vi "Measure vs B2Dv3.vi"() -> ()   [LabVIEW 2009]
doc: "This VI is an example operator panel.\n\nThe VI contains a table for the field values that may be configured manually, or loaded by checking the \"Prompt for File\" box. The data file should contain 3 columns of data, with each column delimited by a tab character.\n\nBefore the VI is executed, set the desired field units and coordinate system. Once the VI is started, follow the directions in the STATUS indicator to operate. Once a field value is achieved, it will be held indefinitely with no user intervention.\n\nThe present field is displayed in the selected units and coordinate system. The present field is queried once per second.\n\nIf a field point is specified that is outside the limits for the magnet, the VI will abort execution."
uses:
  <vilib>/Utility/file.llb/Read From Spreadsheet File (DBL).vi
panel:
  in  "FieldRange":dbl=1.0
  in  "Change\nPID\n(DetermineSIMPID.vi)":bool
  in  "Wait between \nVectors (ms)":u32=4000
  in  "X Axis":enum16{"B", "phi"}(ring)
  in  "Y Axis":T1(ring)=enum."HP (V)"
  out "measured data":dbl[][](array[numeric])
  out "XY Graph":T2(graph)
  in  "Notes:":string="Datum: 22.08.11, Uhrzeit: 18:21, T`0.3K, PID LOOP: P -0.2 I 200 D off, PID Dämpfung: P0,4 D2.2E-5, Laser 25°, 20mA, AOM 10mA, Sweep 0.15T/min " caption="Notizen:"
  out "Messfile Refnum":refnum<file>
  in  "Measurement File":path=path "D:/UserData/Matthias/Messungen/STO_LAOR103/110822/110822_R103_0deg_-0.4--9T_2.txt"
  in  "Sample name:":string="R103"
  in  "HP 1":bool=TRUE
  in  "GPIB HP":string="14"
  in  "LI 4":bool
  in  "GPIB L 4":string="8"
  in  "LI 3":bool
  in  "GPIB L 3":string="8"
  in  "LI 2":bool
  in  "GPIB L 2":string="8"
  in  "LI 1":bool
  in  "GPIB L 1":string="8"
  out "Number of lines":i32=1
  in  "Operation":u16(ring)=1 items=["Stepwise", "Continous"]
  out "Ramp Rate along Vector (T/min)":dbl=0.15000000000000002 format="%.3f"
  out "Current Ramp Rate Z (T/min)":dbl=0.15000000000000002 format="%.3f"
  out "Current Ramp Rate Y (T/min)":dbl format="%.3f"
  in  "User defined Ramp Rate (T/min)":bool=TRUE
  in  "User defined Ramp Rate (T/min)":dbl=0.15 format="%.3f"
  in  "Z-Axis Communications Config":T3={"GPIB address"=22, "GPIB bus"=1, "connection ID"=refnum, "IP"="111.111.111.1", "Active Comm Interface"=0, "Serial Port"="", "Programmer Type"=0} {"Programmer Type" items=["Model 430", "Model 420"]; "Active Comm Interface" items=["TCP/IP (Model 430 Only)", "RS232", "IEEE488"]}
  in  "Max Ramp Rate - Y Axis (A/s)":dbl=0.065 format="%.3f"
  in  "Max Ramp Rate - Z Axis (A/s)":dbl=0.203 format="%.3f"
  in  "Magnitude Limit (kG)":dbl=45.1 format="%.3f"
  in  "Y-Axis Communications Config":T3={"GPIB address"=22, "GPIB bus"=1, "connection ID"=refnum, "IP"="111.111.111.2", "Active Comm Interface"=0, "Serial Port"="", "Programmer Type"=0} {"Programmer Type" items=["Model 430", "Model 420"]; "Active Comm Interface" items=["TCP/IP (Model 430 Only)", "RS232", "IEEE488"]}
  out "Cartesian Display (T)":T4={"Y-Axis Field (T)"=-1e-05, "Z-Axis Field (T)"=-0.15342} {"Z-Axis Field (T)" format="%.3f"; "Y-Axis Field (T)" format="%.3f"}
  in  "Starting index":i32=1
  in  "Normal color":u32(colorbox)=11711154
  in  "Highlight color":u32(colorbox)=16711680
  in  "Prompt for File?":bool
  out "Continue Execution?":bool=TRUE
  out "error out":T5
  in  "error in":T5
  out "STATUS":string="Holding at current vector. Set Ramping Mode to NEXT VECTOR to continue."
  in  "Ramping Control":u16(ring)=2 items=["NEXT VECTOR", "RAMPING", "HOLDING", "PAUSE", "ZERO"]
  out "Cartesian Display (kG)":T6 {"Z-Axis Field (kG)" format="%.3f"; "Y-Axis Field (kG)" format="%.3f"}
  in  "Field Values":string[][](table)=[["0", "-0.4"]]
  out "Switch Heaters":bool=TRUE
  out "Polar Display (T)":T7={"q (degrees)"=90.0, "Field Magnitude (T)"=2e-05} {"Field Magnitude (T)" format="%.3f"; "q (degrees)" format="%.3f"}
  out "Polar Display (kG)":T8 {"Field Magnitude (kG)" format="%.3f"; "q (degrees)" format="%.3f"}
  in  "Coordinate System":u16(ring) items=["Cartesian", "Polar"]
  in  "Magnetic Field Units":u16(ring)=1 items=["kG", "Tesla"]
  # "Measurement Display"
  # "Measurement Settings"
  # "Magnet Settings"
  # "Max Ramp Rate z: 1.27 T/min\nMax Ramp Rate y: 0.17 T/min"
  # "Devices"
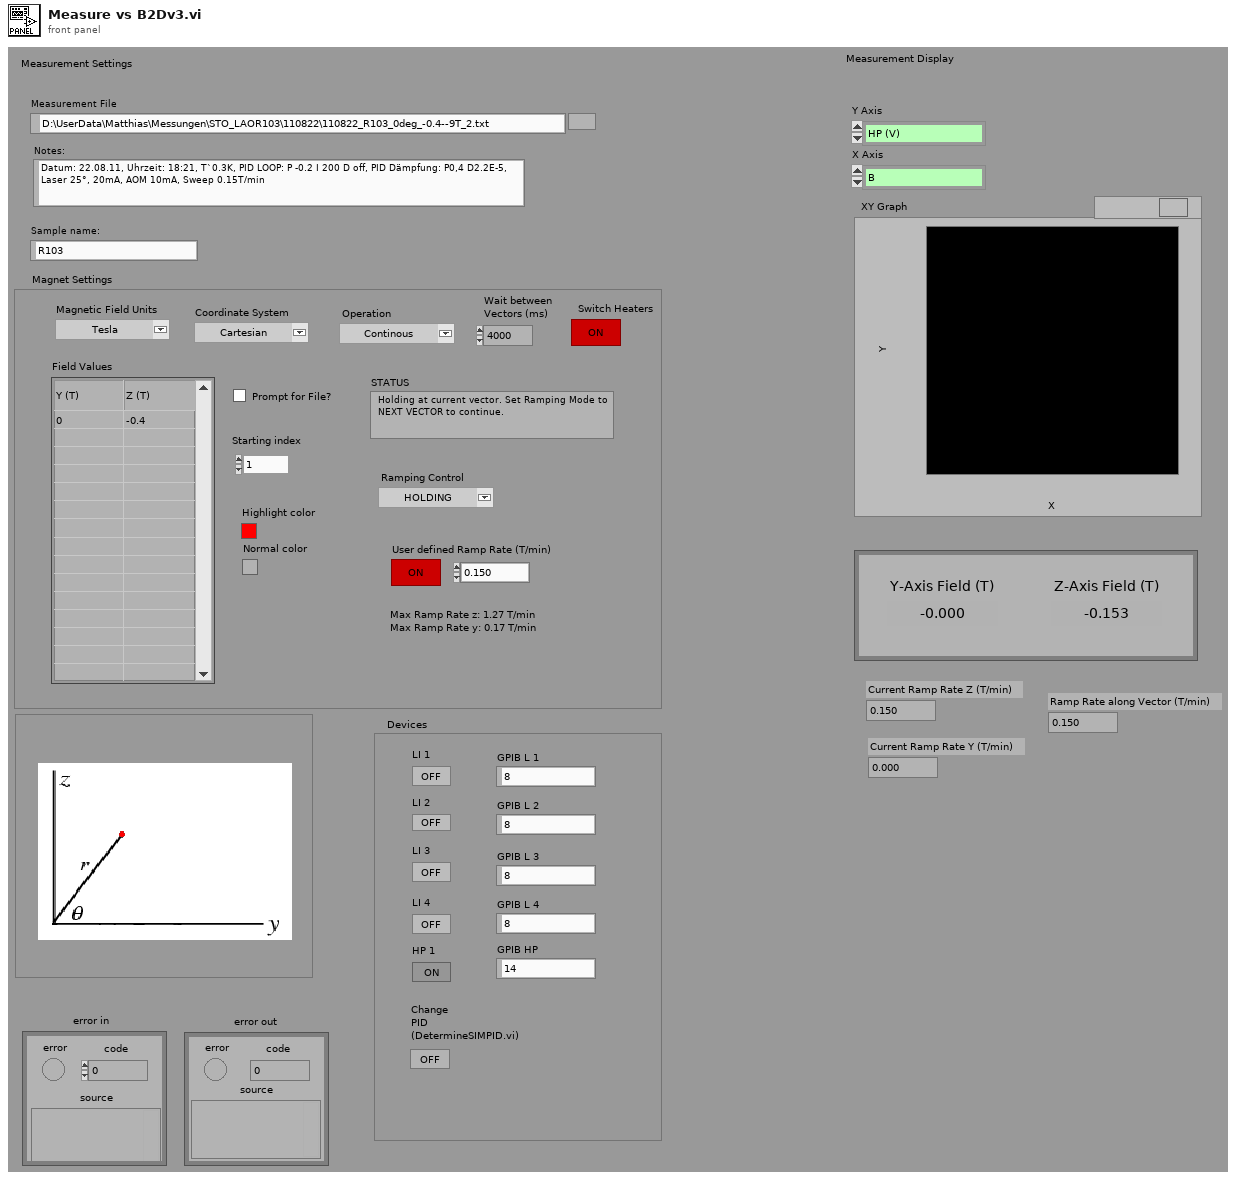
[diagram p1: front panel]
types:
  T1 = enum16{"B", "phi", "LI 1 Vx", "LI 1 phase", "LI 2 Vx", "LI 2 phase", "LI 3 Vx", "LI 3 phase", "LI 4 Vx", "LI 4 phase", "HP (V)"}
  T2 = cluster{"measured data":dbl[], "measured data":dbl[]}
  T3 = cluster{"GPIB address":i16, "GPIB bus":i16, "connection ID":refnum<k5>, "IP":string, "Active Comm Interface":u16, "Serial Port":refnum<visa-resource-name>, "Programmer Type":u16}
  T4 = cluster{"Y-Axis Field (T)":dbl, "Z-Axis Field (T)":dbl}
  T5 = cluster{"error":bool, "code":i32, "source":string}
  T6 = cluster{"Y-Axis Field (kG)":dbl, "Z-Axis Field (kG)":dbl}
  T7 = cluster{"q (degrees)":dbl, "Field Magnitude (T)":dbl}
  T8 = cluster{"q (degrees)":dbl, "Field Magnitude (kG)":dbl}
  T9 = enum16{"", "RAMPING", "HOLDING", "PAUSED", "MANUAL UP", "MANUAL DOWN", "ZEROING CURRENT", "QUENCH DETECTED", "HEATING SWITCH"}
  T10 = enum16{"", "RAMPING", "HOLDING", "PAUSED", "MANUAL UP", "MANUAL DOWN", "ZEROING CURRENT", "QUENCH DETECTED", "HEATING SWITCH", "AT ZER0", "COOLING SWITCH"}
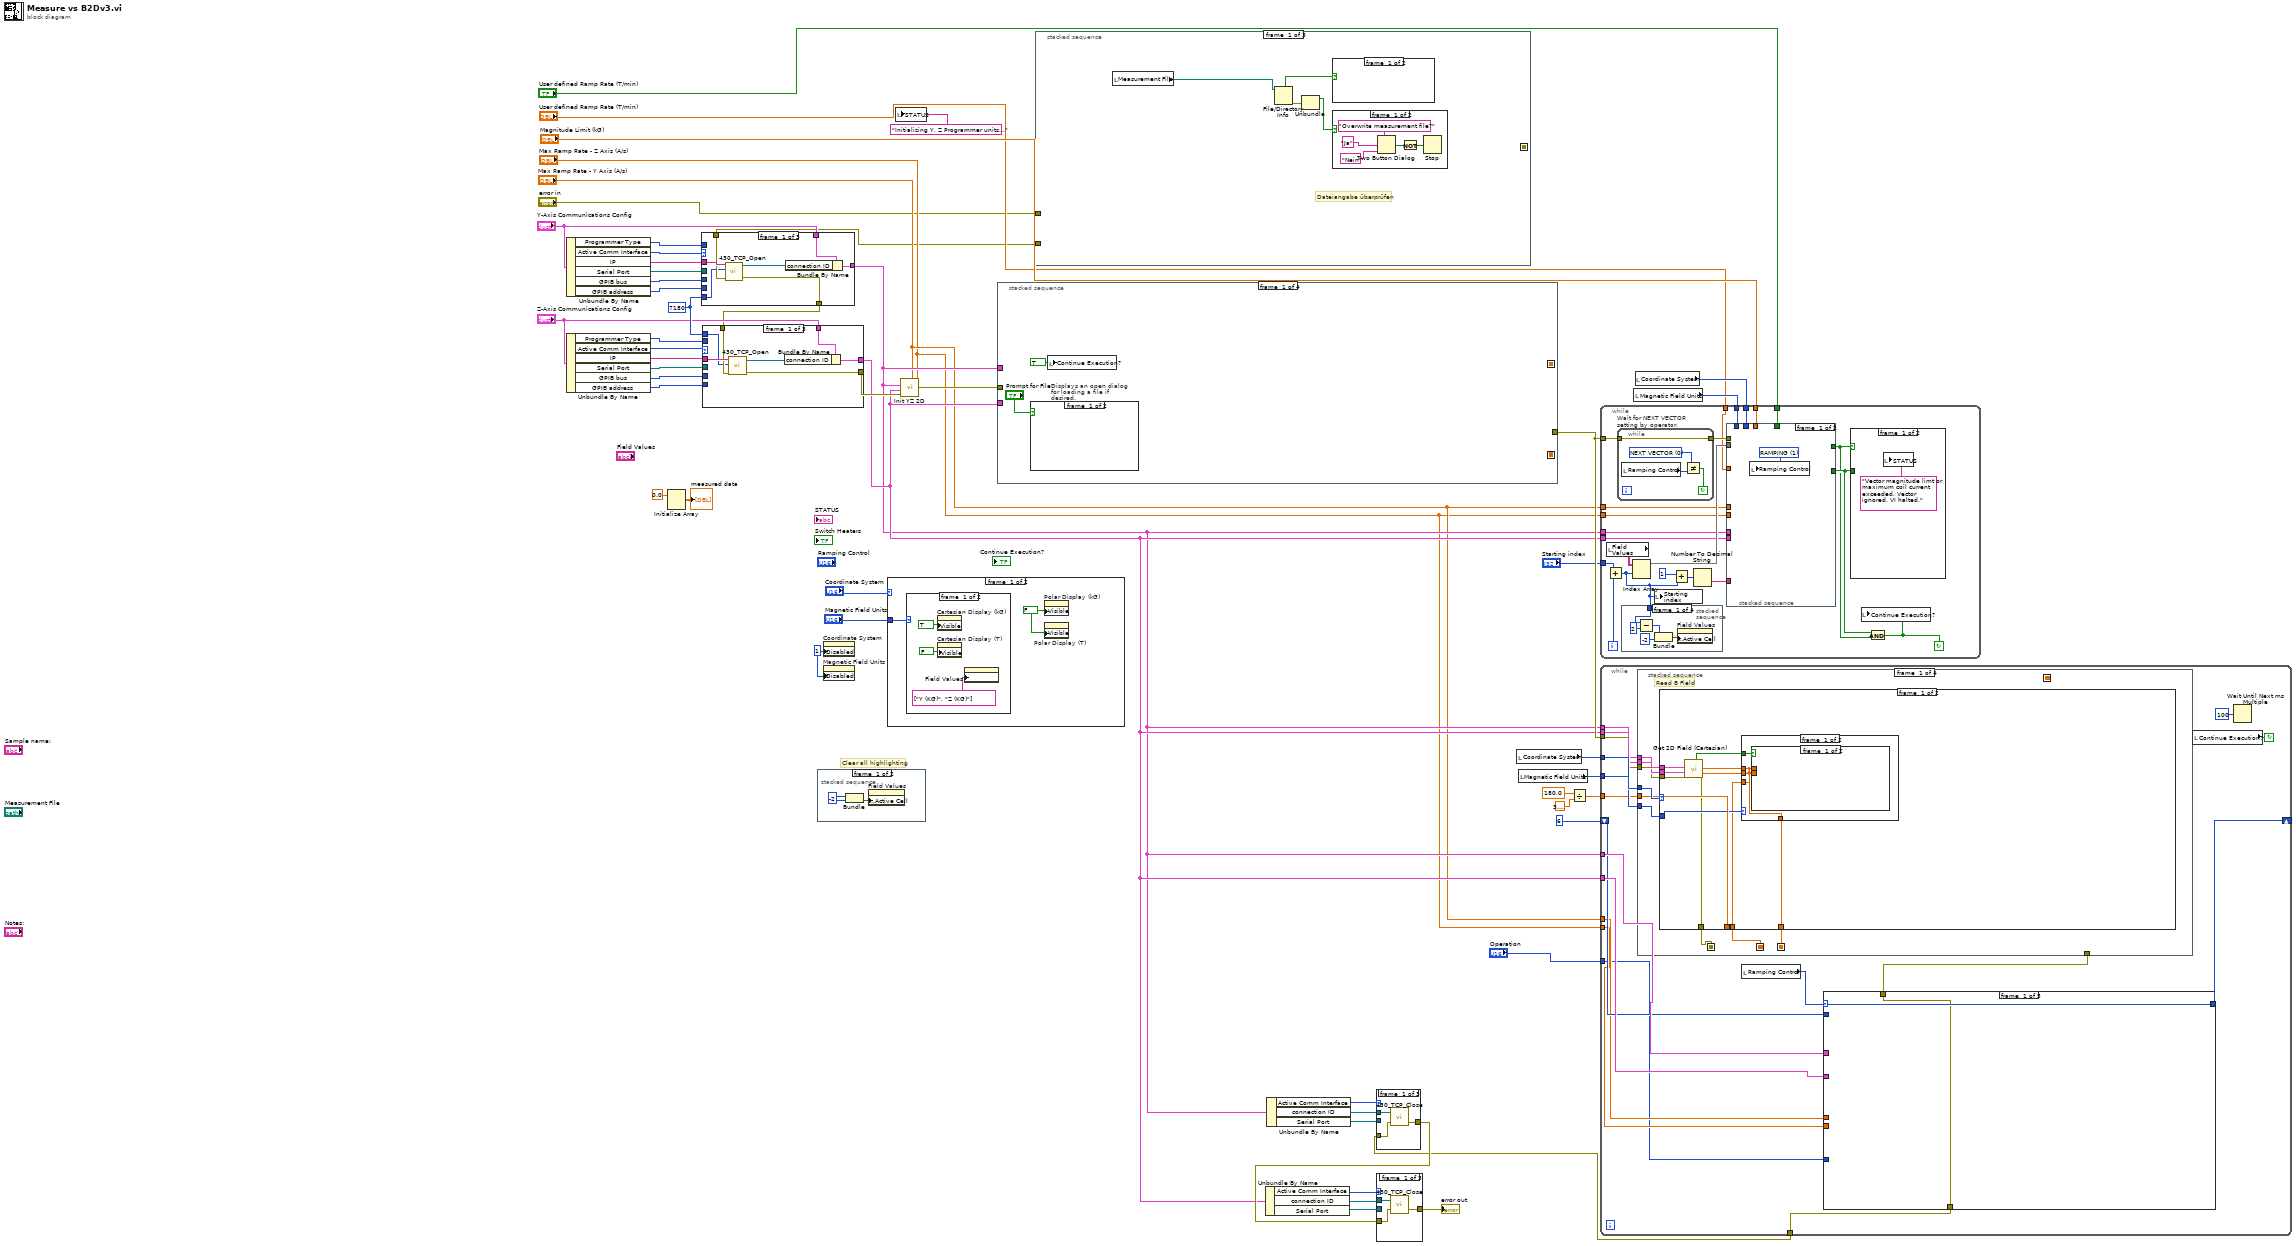
[diagram p0: block diagram]
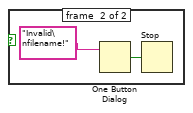
[diagram p3: hidden frame]
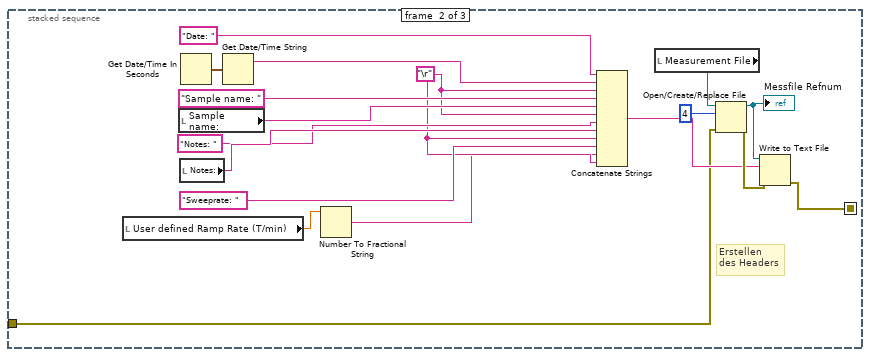
[diagram p4: hidden frame]
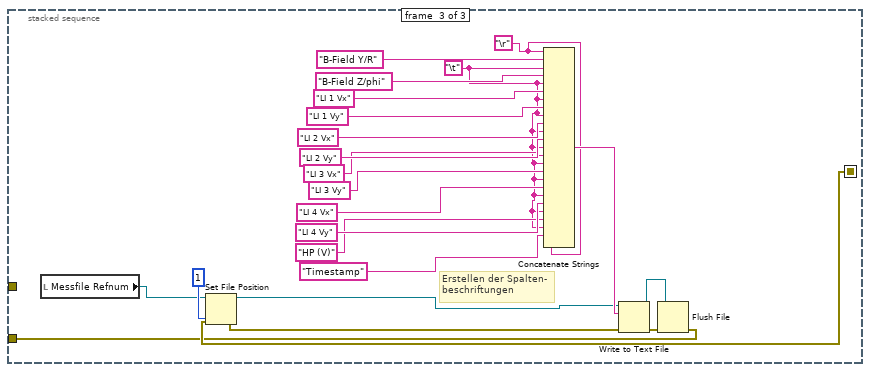
[diagram p5: hidden frame]
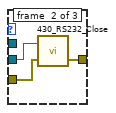
[diagram p6: hidden frame]
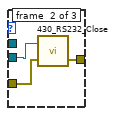
[diagram p8: hidden frame]
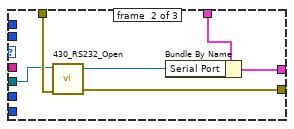
[diagram p10: hidden frame]
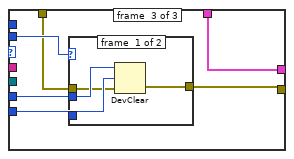
[diagram p11: hidden frame]
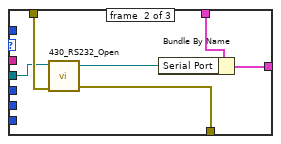
[diagram p13: hidden frame]
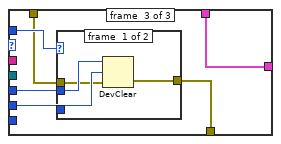
[diagram p14: hidden frame]
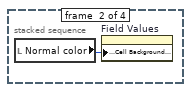
[diagram p16: hidden frame]
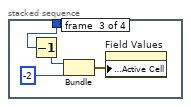
[diagram p17: hidden frame]
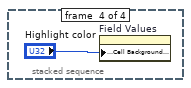
[diagram p18: hidden frame]
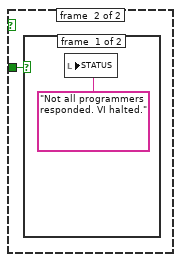
[diagram p19: hidden frame]
diagram:
  w38 = 7180 ("TCP Port")
  w51 = u8 1 ("Write Attribute")
  # "Clear all highlighting"
  n1 = Unbundle By Name("Z-Axis Communications Config") -> ("Programmer Type"=w14:u16, "Active Comm Interface"=w37:u16, "IP"=w34:string, "Serial Port"=w33:refnum<visa-resource-name>, "GPIB bus"=w13:i16, "GPIB address"=w12:i16)
  n2 = Unbundle By Name("Y-Axis Communications Config") -> ("Programmer Type"=w8:u16, "Active Comm Interface"=w36:u16, "IP"=w35:string, "Serial Port"=w32:refnum<visa-resource-name>, "GPIB bus"=w9:i16, "GPIB address"=w10:i16)
  n3 = Initialize Array(0.0 ("element")) -> (→"measured data":dbl[][])  [unwired: 2 in]
  n4 = stacked-sequence {
    frame #0 {
      w54 = -2
      n5 = Bundle(w54, w54) -> (w55:cluster{i32, i32})  [unwired: 1 in]
      n6 = property on="Field Values" class="Tbl (strict)"("Active Cell:Active Cell"=w55) -> ()  [unwired: 2 in, 2 out]
    }
    frame #1 {
      n7 = property on="Field Values" class="Tbl (strict)"("Active Cell:Cell Background Color"="Normal color") -> ()  [unwired: 2 in, 2 out]
    }
  }
  n8 = property on="Coordinate System" class="Ring (strict)"("Disabled"=w51) -> ()  [unwired: 2 in, 2 out]
  n9 = property on="Magnetic Field Units" class="Ring (strict)"("Disabled"=w51) -> ()  [unwired: 2 in, 2 out]
  n10 = case shown="0, Default" "Coordinate System" {
    tunnel: "Magnetic Field Units" -> [w58 w66]
    frame #0 {
      w57 = FALSE ("Write Attribute")
      (unwired) FALSE ("Write Attribute")
      (unwired) TRUE ("Write Attribute")
      n11 = case shown="1" w58 {
        frame #0 {
          n12 = property on="Cartesian Display (kG)" class="Cluster (strict)"("Visible"=TRUE ("Write Attribute")) -> ()  [unwired: 2 in, 2 out]
          n13 = property on="Cartesian Display (T)" class="Cluster (strict)"("Visible"=FALSE ("Write Attribute")) -> ()  [unwired: 2 in, 2 out]
          n14 = property on="Field Values" class="Tbl (strict)"("Column Header Strings[]"=string[] ["Y (KG)", "Z (KG)"] ("Write Attribute")) -> ()  [unwired: 2 in, 2 out]
        }
        frame #1 {
          n15 = property on="Cartesian Display (kG)" class="Cluster (strict)"("Visible"=FALSE ("Write Attribute")) -> ()  [unwired: 2 in, 2 out]
          n16 = property on="Cartesian Display (T)" class="Cluster (strict)"("Visible"=TRUE ("Write Attribute")) -> ()  [unwired: 2 in, 2 out]
          n17 = property on="Field Values" class="Tbl (strict)"("Column Header Strings[]"=string[] ["Y (T)", "Z (T)"] ("Write Attribute")) -> ()  [unwired: 2 in, 2 out]
        }
      }
      n18 = property on="Polar Display (kG)" class="Clust (strict)"("Visible"=w57) -> ()  [unwired: 2 in, 2 out]
      n19 = property on="Polar Display (T)" class="Clust (strict)"("Visible"=w57) -> ()  [unwired: 2 in, 2 out]
    }
    frame #1 {
      (unwired) FALSE ("Write Attribute")
      (unwired) TRUE ("Write Attribute")
      w65 = FALSE ("Write Attribute")
      n20 = case shown="1" w66 {
        frame #0 {
          n21 = property on="Polar Display (kG)" class="Clust (strict)"("Visible"=TRUE ("Write Attribute")) -> ()  [unwired: 2 in, 2 out]
          n22 = property on="Polar Display (T)" class="Clust (strict)"("Visible"=FALSE ("Write Attribute")) -> ()  [unwired: 2 in, 2 out]
          n23 = property on="Field Values" class="Tbl (strict)"("Column Header Strings[]"=string[] ["Mag. r (KG)", "Theta (deg)"] ("Write Attribute")) -> ()  [unwired: 2 in, 2 out]
        }
        frame #1 {
          n24 = property on="Polar Display (kG)" class="Clust (strict)"("Visible"=FALSE ("Write Attribute")) -> ()  [unwired: 2 in, 2 out]
          n25 = property on="Polar Display (T)" class="Clust (strict)"("Visible"=TRUE ("Write Attribute")) -> ()  [unwired: 2 in, 2 out]
          n26 = property on="Field Values" class="Tbl (strict)"("Column Header Strings[]"=string[] ["Mag. r (T)", "Theta (deg)"] ("Write Attribute")) -> ()  [unwired: 2 in, 2 out]
        }
      }
      n27 = property on="Cartesian Display (kG)" class="Cluster (strict)"("Visible"=w65) -> ()  [unwired: 2 in, 2 out]
      n28 = property on="Cartesian Display (T)" class="Cluster (strict)"("Visible"=w65) -> ()  [unwired: 2 in, 2 out]
    }
  }
  n29 = local write "STATUS"("Initializing Y, Z Programmer units..." ("STATUS")) -> ()
  n30 = stacked-sequence {
    seq-local: [_ w84 _] -> [_ _ w103]
    tunnel: "error in" -> [_ w85 _]
    tunnel: [_ _ w102] -> w3
    frame #0 {
      # "Dateiangabe überprüfen"
      n31 = local read "Measurement File"() -> (w76:path)
      n32 = File/Directory Info(path=w76) -> (directory=w74:bool, error out=w75:errorcluster)  [unwired: 1 in, 5 out]
      n33 = Unbundle(w75) -> ("status"=w73:bool)  [unwired: 2 out]
      n34 = case shown="False" w74 {
        frame #0 {
        }
        frame #1 {
          n35 = One Button Dialog(message="Invalid\nfilename!") -> (true=w82:bool)  [unwired: 1 in]
          n36 = Stop(stop? (T)=w82) -> ()
        }
      }
      n37 = case shown="False" w73 {
        frame #0 {
          n38 = Two Button Dialog(message="Overwrite measurement file?", 1:"Nein", 2:"Ja") -> (T button?=w78:bool)
          n39 = Not(x=w78) -> (.not. x?=w77:bool)
          n40 = Stop(stop? (T)=w77) -> ()
        }
        frame #1 {
        }
      }
    }
    frame #1 {
      w88 = "\r"
      # "Erstellen\ndes Headers"
      n41 = local read "User defined Ramp Rate (T/min)"() -> (w87:dbl)
      n42 = local read "Sample name:"() -> (w94:string)
      n43 = local read "Notes:"() -> (w96:string)
      n44 = Get Date/Time In Seconds() -> (seconds since 1Jan1904=w90:timestamp)
      n45 = Get Date/Time String(seconds (now)=w90) -> (date string=w92:string)  [unwired: 2 in, 1 out]
      n46 = Number To Fractional String(number=w87) -> (F-format string=w86:string)  [unwired: 3 in]
      n47 = Concatenate Strings("Date: ", w92, w88, "Sample name: ", w94, w88, "Notes: ", w96, w88, "Sweeprate: ", w86, w88) -> (w100:string)
      n48 = local read "Measurement File"() -> (w97:path)
      n49 = Open/Create/Replace File(file path (use dialog)=w97, error in=w85, operation (0:open)=4) -> (refnum out=w99:refnum<file>, error out=w101:errorcluster)  [unwired: 3 in, 1 out]
      "Messfile Refnum" <- w99
      n50 = Write to Text File(file (use dialog)=w99, text=w100, error in=w101) -> (error out=w84:errorcluster)  [unwired: 1 in, 2 out]
    }
    frame #2 {
      w106 = "\t"
      w104 = "\r"
      # "Erstellen der Spalten-\nbeschriftungen"
      n51 = local read "Messfile Refnum"() -> (w113:refnum<file>)
      n52 = Set File Position(refnum=w113, from (0:start)=1, error in=w103) -> (refnum out=w119:refnum<file>, error out=w121:errorcluster)  [unwired: 1 in]
      n53 = Concatenate Strings(w104, "B-Field Y/R", w106, "B-Field Z/phi", w106, "LI 1 Vx", w106, "LI 1 Vy", w106, "LI 2 Vx", w106, "LI 2 Vy", w106, "LI 3 Vx", w106, "LI 3 Vy", w106, "LI 4 Vx", w106, "LI 4 Vy", w106, "HP (V)", w106, "Timestamp", w104) -> (w120:string)
      n54 = Write to Text File(file (use dialog)=w119, text=w120, error in=w121) -> (refnum out=w123:refnum<file>, error out=w122:errorcluster)  [unwired: 1 in, 1 out]
      n55 = Flush File(refnum=w123, error in=w122) -> (error out=w102:errorcluster)  [unwired: 1 out]
    }
  }
  n56 = case shown="2" w36 {
    tunnel: w35 -> [w131 _ _]
    tunnel: w3 -> [w130 w137 w139]
    tunnel: "Y-Axis Communications Config" -> [w129 w132 w143]
    tunnel: [w127 w135 w143] -> w21
    tunnel: [w126 w136 w138] -> w11
    tunnel: w38 -> [w125 _ _]
    tunnel: w32 -> [_ w133 _]
    tunnel: w10 -> [_ _ w142]
    tunnel: w9 -> [_ _ w141]
    tunnel: w8 -> [_ _ w140]
    frame #0 {
      n57 = call <userlib>:"430_TCP_Open.vi"("IP Address"=w131, "TCP Port"=w125, "error in (no error)"=w130) -> ("connection ID"=w128:refnum<k5>, "error out"=w126:errorcluster)  [unwired: 3 in, 1 out]
      n58 = Bundle By Name(cluster=w129, "connection ID"=w128) -> (w127:T3)
    }
    frame #1 {
      n59 = call <userlib>:"430_RS232_Open.vi"("VISA resource name"=w133, "error in (no error)"=w137) -> ("VISA resource name out"=w134:refnum<visa-resource-name>, "error out"=w136:errorcluster)  [unwired: 5 in]
      n60 = Bundle By Name(cluster=w132, "Serial Port"=w134) -> (w135:T3)
    }
    frame #2 {
      n61 = case shown="0, Default" w140 {
        tunnel: w141 -> [w147 _]
        tunnel: w142 -> [w146 _]
        tunnel: w139 -> [w145 w148]
        tunnel: [w144 w148] -> w138
        frame #0 {
          n62 = DevClear(2:w145, 3:w146, 4:w147) -> (0:w144:errorcluster)  [unwired: 1 out]
        }
        frame #1 {
        }
      }
    }
  }
  n63 = case shown="2" w37 {
    tunnel: w34 -> [w155 _ _]
    tunnel: w11 -> [w154 w161 w163]
    tunnel: [w153 w160 w162] -> w31
    tunnel: "Z-Axis Communications Config" -> [w152 w158 w167]
    tunnel: [w150 w159 w167] -> w22
    tunnel: w38 -> [w149 _ _]
    tunnel: w33 -> [_ w156 _]
    tunnel: w14 -> [_ _ w166]
    tunnel: w13 -> [_ _ w165]
    tunnel: w12 -> [_ _ w164]
    frame #0 {
      n64 = call <userlib>:"430_TCP_Open.vi"("IP Address"=w155, "TCP Port"=w149, "error in (no error)"=w154) -> ("connection ID"=w151:refnum<k5>, "error out"=w153:errorcluster)  [unwired: 3 in, 1 out]
      n65 = Bundle By Name(cluster=w152, "connection ID"=w151) -> (w150:T3)
    }
    frame #1 {
      n66 = call <userlib>:"430_RS232_Open.vi"("VISA resource name"=w156, "error in (no error)"=w161) -> ("VISA resource name out"=w157:refnum<visa-resource-name>, "error out"=w160:errorcluster)  [unwired: 5 in]
      n67 = Bundle By Name(cluster=w158, "Serial Port"=w157) -> (w159:T3)
    }
    frame #2 {
      n68 = case shown="0, Default" w166 {
        tunnel: w165 -> [w171 _]
        tunnel: w164 -> [w170 _]
        tunnel: w163 -> [w169 w172]
        tunnel: [w168 w172] -> w162
        frame #0 {
          n69 = DevClear(2:w169, 3:w170, 4:w171) -> (0:w168:errorcluster)  [unwired: 1 out]
        }
        frame #1 {
        }
      }
    }
  }
  n70 = call <userlib>:"Init YZ 2D.vi"("Max Ramp Rate Z-axis"="Max Ramp Rate - Z Axis (A/s)", "Max Ramp Rate Y-axis"="Max Ramp Rate - Y Axis (A/s)", "error in"=w31, "Z-Axis Communications Config"=w22, "Y-Axis Communications Config"=w21) -> ("error out"=w49:T5)  [unwired: 5 in]
  n71 = stacked-sequence {
    seq-local: [_ w180 _ _] -> [_ _ w227 _]
    seq-local: [_ w179 _ _] -> [_ _ w226 _]
    tunnel: w22 -> [_ w182 _ _]
    tunnel: w49 -> [_ w183 _ _]
    tunnel: [_ w178 _ _] -> w45
    tunnel: w21 -> [_ w181 _ _]
    frame #0 {
      n72 = case "Displays an open dialog for loading a file if desired." shown="True" "Prompt for File?" {
        frame #0 {
        }
        frame #1 {
          n73 = call-poly <vilib>:"Read From Spreadsheet File.vi"() -> ("all rows"=w177:dbl[][])  [unwired: 7 in, 4 out]
          n74 = Number To Fractional String(number=w177, precision (6)=i16 4) -> (F-format string=w176:string[][])  [unwired: 2 in]
          n75 = local write "Field Values"(w176) -> ()
        }
      }
      n76 = local write "Continue Execution?"(TRUE ("Continue Execution?")) -> ()
    }
    frame #1 {
      w191 = u16 3 items=["NEXT VECTOR", "RAMPING", "HOLDING", "PAUSE", "ZERO"] ("Ramping Control")
      n77 = call <userlib>:"Get Switch Present.vi"("error in"=w183, "Communications Config"=w181) -> ("error out"=w187:T5, "Switch Present?"=w188:bool)
      n78 = case shown="True" w188 {
        tunnel: w187 -> [w209 w218]
        tunnel: w181 -> [_ w211]
        tunnel: [0.0 w215] -> w179
        tunnel: [w209 w217] -> w186
        frame #0 {
        }
        frame #1 {
          n79 = call <userlib>:"Get Switch Heater Time.vi"("error in"=w218, "Communications Config"=w211) -> ("error out"=w214:T5, "Switch Heating Time (secs)"=w216:dbl)
          n80 = call <userlib>:"Get Switch Heater.vi"("error in"=w214, "Communications Config"=w211) -> ("error out"=w213:T5, "Switch Heater Indicator"=w212:bool)
          n81 = case shown="False" w212 {
            tunnel: [w223 w224] -> w217
            tunnel: w216 -> [w221 _]
            tunnel: [w221 0.0] -> w215
            tunnel: w213 -> [w219 w224]
            tunnel: w211 -> [w220 _]
            frame #0 {
              n82 = call <userlib>:"Set Switch Heater.vi"("error in"=w219, "Switch Heater Control"=TRUE, "Communications Config"=w220) -> ("error out"=w223:T5)
            }
            frame #1 {
            }
          }
        }
      }
      n83 = call <userlib>:"Get Switch Present.vi"("error in"=w186, "Communications Config"=w182) -> ("error out"=w184:T5, "Switch Present?"=w185:bool)
      n84 = case shown="True" w185 {
        tunnel: w184 -> [w192 w201]
        tunnel: w182 -> [_ w194]
        tunnel: [0.0 w198] -> w180
        tunnel: [w192 w200] -> w178
        frame #0 {
        }
        frame #1 {
          n85 = call <userlib>:"Get Switch Heater Time.vi"("error in"=w201, "Communications Config"=w194) -> ("error out"=w197:T5, "Switch Heating Time (secs)"=w199:dbl)
          n86 = call <userlib>:"Get Switch Heater.vi"("error in"=w197, "Communications Config"=w194) -> ("error out"=w196:T5, "Switch Heater Indicator"=w195:bool)
          n87 = case shown="False" w195 {
            tunnel: [w202 w207] -> w200
            tunnel: w199 -> [w205 _]
            tunnel: [w205 0.0] -> w198
            tunnel: w196 -> [w203 w207]
            tunnel: w194 -> [w204 _]
            frame #0 {
              n88 = call <userlib>:"Set Switch Heater.vi"("error in"=w203, "Switch Heater Control"=TRUE, "Communications Config"=w204) -> ("error out"=w202:T5)
            }
            frame #1 {
            }
          }
        }
      }
      n89 = local write "Ramping Control"(w191) -> ()
      n90 = local write "Switch Heaters"(TRUE ("Switch Heater Control")) -> ()
      n91 = property on="Switch Heaters" class="Boolean (strict)"("Disabled"=u8 1 ("Write Attribute")) -> ()  [unwired: 2 in, 2 out]
    }
    frame #2 {
      n92 = Max & Min(x=w227, y=w226) -> (max(x,y)=w228:dbl)  [unwired: 1 out]
      n93 = local write "STATUS"("Heating switches..." ("STATUS")) -> ()
      n94 = Add(x=w228, y=2) -> (x+y=w232:dbl)
      n95 = property on="Ramping Control" class="Ring (strict)"("Disabled"=u8 1 ("Write Attribute")) -> ()  [unwired: 2 in, 2 out]
      n96 = Multiply(x=w232, y=1000) -> (x*y=w231:dbl)
      n97 = Wait (ms)(milliseconds to wait=w231) -> ()  [unwired: 1 out]
    }
    frame #3 {
      n98 = property on="Ramping Control" class="Ring (strict)"("Disabled"=u8 0 ("Write Attribute")) -> ()  [unwired: 2 in, 2 out]
      n99 = local write "STATUS"("Ready to ramp to first vector. Set Ramping Mode to NEXT VECTOR to begin." ("STATUS")) -> ()
      n100 = local read "Field Values"() -> (w237:string[][])
      n101 = Array Size(array=w237) -> (size(s)=w236:i32[])
      n102 = Index Array(array=w236, index=0) -> (element=→"Number of lines":i32)
    }
  }
  n103 = Unbundle By Name(w22) -> ("Active Comm Interface"=w28:u16, "connection ID"=w27:refnum<k5>, "Serial Port"=w26:refnum<visa-resource-name>)
  n104 = Unbundle By Name(w21) -> ("Active Comm Interface"=w29:u16, "connection ID"=w25:refnum<k5>, "Serial Port"=w24:refnum<visa-resource-name>)
  n105 = local read "Coordinate System"() -> (w46:u16)
  n106 = local read "Magnetic Field Units"() -> (w44:u16)
  n107 = Divide(x=180.0, y=3.141592653589793) -> (x/y=w41:dbl)
  n108 = while {
    shift-left: u16 6 ("Ramping Control") -> [w245]
    shift-right: [w246] -> _
    tunnel: [w248] -> w23
    tunnel: w22 -> [w249]
    tunnel: w21 -> [w250]
    tunnel: w41 -> [w252]
    tunnel: w44 -> [w253]
    tunnel: w45 -> [w254]
    tunnel: w22 -> [w255]
    tunnel: w21 -> [w256]
    tunnel: w46 -> [w257]
    tunnel: "Max Ramp Rate - Y Axis (A/s)" -> [w244]
    tunnel: "Max Ramp Rate - Z Axis (A/s)" -> [w243]
    tunnel: "Operation" -> [w242]
    stop <- w247 continue-if-true
    n109 = stacked-sequence {
      seq-local: [w261 _ _ _] -> [_ _ w361 _]
      seq-local: [w260 _ _ _] -> [_ w330 w355 _]
      seq-local: [w259 _ _ _] -> [_ _ w356 _]
      seq-local: [_ _ w342 _] -> [_ _ _ w422]
      tunnel: w257 -> [w267 _ _ w420]
      tunnel: w256 -> [w266 _ _ _]
      tunnel: w255 -> [w265 _ _ _]
      tunnel: w254 -> [w264 _ _ _]
      tunnel: w253 -> [w263 _ _ _]
      tunnel: w252 -> [w262 _ _ _]
      tunnel: [_ _ w357 _] -> w241
      frame #0 {
        # "Read B Field"
        n110 = case shown="0, Default" w267 {
          tunnel: w266 -> [w277 w300]
          tunnel: w265 -> [w276 w299]
          tunnel: w264 -> [w275 w298]
          tunnel: w263 -> [w274 w297]
          tunnel: w262 -> [_ w296]
          tunnel: [w270 w295] -> w261
          tunnel: [w269 w293] -> w260
          tunnel: [w268 w294] -> w259
          frame #0 {
            n111 = call <userlib>:"Get 2D Field (Cartesian).vi"("Y-Axis Communications Config"=w277, "Z-Axis Communications Config"=w276, "error in"=w275) -> ("All Instruments Responded?"=w271:bool, "Y-Axis Field (kG)"=w273:dbl, "Z-Axis Field (kG)"=w272:dbl, "error out"=w270:T5)  [unwired: 2 in]
            n112 = case shown="1" w274 {
              tunnel: w273 -> [w278 w286]
              tunnel: w272 -> [w279 w287]
              tunnel: w271 -> [w280 w289]
              tunnel: [w279 w285] -> w269
              tunnel: [w278 w284] -> w268
              frame #0 {
                n113 = case shown="True" w280 {
                  tunnel: w278 -> [_ w282]
                  tunnel: w279 -> [_ w281]
                  frame #0 {
                  }
                  frame #1 {
                    n114 = Bundle("Y-Axis Field (kG)"=w282, "Z-Axis Field (kG)"=w281) -> (→"Cartesian Display (kG)":T6)  [unwired: 1 in]
                  }
                }
              }
              frame #1 {
                w288 = 0.1 ("y")
                n115 = Multiply(x=w286, y=w288) -> (x*y=w284:dbl)
                n116 = Multiply(x=w287, y=w288) -> (x*y=w285:dbl)
                n117 = case shown="True" w289 {
                  tunnel: w284 -> [_ w292]
                  tunnel: w285 -> [_ w291]
                  frame #0 {
                  }
                  frame #1 {
                    n118 = Bundle(w292, w291) -> (→"Cartesian Display (T)":cluster{dbl, dbl})  [unwired: 1 in]
                  }
                }
              }
            }
          }
          frame #1 {
            n119 = stacked-sequence {
              tunnel: w300 -> [w311]
              tunnel: w299 -> [w310]
              tunnel: w298 -> [w309]
              tunnel: w297 -> [w308]
              tunnel: w296 -> [w305]
              tunnel: [w303] -> w295
              tunnel: [w302] -> w294
              tunnel: [w301] -> w293
              frame #0 {
                # "Field"
                n120 = call <userlib>:"Get 2D Field (Polar).vi"("Y-Axis Communications Config"=w311, "Z-Axis Communications Config"=w310, "error in"=w309) -> ("All Instruments Responded?"=w304:bool, "Radial (r) Field (kG)"=w307:dbl, "q (radians)"=w306:dbl, "error out"=w303:T5)  [unwired: 2 in]
                n121 = case shown="0, Default" w308 {
                  tunnel: w307 -> [w313 w325]
                  tunnel: w306 -> [w315 w324]
                  tunnel: w305 -> [w314 w323]
                  tunnel: w304 -> [w316 w322]
                  tunnel: [w313 w320] -> w302
                  tunnel: [w312 w321] -> w301
                  frame #0 {
                    n122 = Multiply(x=w315, y=w314) -> (x*y=w312:dbl)
                    n123 = case shown="True" w316 {
                      tunnel: w313 -> [_ w317]
                      tunnel: w312 -> [_ w318]
                      frame #0 {
                      }
                      frame #1 {
                        n124 = Bundle(w318, "Radial (r) Field (kG)"=w317) -> (→"Polar Display (kG)":cluster{dbl, "Radial (r) Field (kG)":dbl})  [unwired: 1 in]
                      }
                    }
                  }
                  frame #1 {
                    n125 = Multiply(x=w325, y=0.1) -> (x*y=w321:dbl)
                    n126 = Multiply(x=w324, y=w323) -> (x*y=w320:dbl)
                    n127 = case shown="True" w322 {
                      tunnel: w321 -> [_ w327]
                      tunnel: w320 -> [_ w328]
                      frame #0 {
                      }
                      frame #1 {
                        n128 = Bundle(w328, w327) -> (→"Polar Display (T)":cluster{dbl, dbl})  [unwired: 1 in]
                      }
                    }
                  }
                }
              }
            }
          }
        }
      }
      frame #1 {
        # "Change PID"
        n129 = case shown="True" "Change\nPID\n(DetermineSIMPID.vi)" {
          tunnel: w330 -> [_ w335]
          frame #0 {
          }
          frame #1 {
            # "z Field Value"
            n130 = call "CheckFieldRange.vi"("Field Value"=w335) -> ("Field Range"=w332:dbl)  [unwired: 10 in]
            n131 = Equal?(x="FieldRange", y=w332) -> (x = y?=w334:bool)
            n132 = case shown="False" w334 {
              tunnel: w332 -> [w340 w341]
              frame #0 {
                n133 = local write "FieldRange"(w340) -> ()
                n134 = call "DetermineSIMPID.vi"("Field Range"=w340) -> ("D"=w338:string, "P"=w339:string)  [unwired: 7 in, 2 out]
                n135 = call "SIM960ChangeP.vi"("New D Value"=w338, "New P Value"=w339, "Port Num- PID"="1", "GPIB-Adress"="2") -> ()  [unwired: 8 in]
              }
              frame #1 {
                n136 = local write "FieldRange"(w341) -> ()
              }
            }
          }
        }
      }
      frame #2 {
        # "Zeile in Datei schreiben"
        # "Read and Save Devices"
        n137 = stacked-sequence {
          tunnel: [w366 _ _ _ _ _] -> w354
          tunnel: [w365 _ _ _ _ _] -> w353
          tunnel: [_ w379 _ _ _ _] -> w350
          tunnel: [_ w377 _ _ _ _] -> w349
          tunnel: [_ _ w389 _ _ _] -> w348
          tunnel: [_ _ w388 _ _ _] -> w347
          tunnel: [_ _ _ w400 _ _] -> w346
          tunnel: [_ _ _ w399 _ _] -> w345
          tunnel: [_ _ _ _ w410 _] -> w344
          tunnel: [_ _ _ _ _ w416] -> w343
          frame #0 {
            n138 = case shown="True" "LI 1" {
              tunnel: ["0" ("Antwort2") w373] -> w368
              tunnel: ["0" ("Antwort1") w372] -> w367
              frame #0 {
              }
              frame #1 {
                n139 = call "LI-Ansteuerung.vi"("Frage2"="OUTP? 4", "Frage1"="OUTP? 1", "address string"="GPIB L 1") -> ("Antwort2"=w373:string, "Antwort1"=w372:string)
              }
            }
            n140 = Fract/Exp String To Number(string=w368) -> (number=w365:dbl)  [unwired: 3 in, 1 out]
            n141 = Fract/Exp String To Number(string=w367) -> (number=w366:dbl)  [unwired: 3 in, 1 out]
          }
          frame #1 {
            n142 = case shown="False" "LI 2" {
              tunnel: [w382 w384] -> w378
              tunnel: [w382 w383] -> w380
              frame #0 {
                w382 = "0" ("Antwort1")
              }
              frame #1 {
                n143 = call "LI-Ansteuerung.vi"("Frage2"="OUTP? 4", "Frage1"="OUTP? 1", "address string"="GPIB L 2") -> ("Antwort2"=w384:string, "Antwort1"=w383:string)
              }
            }
            n144 = Fract/Exp String To Number(string=w378) -> (number=w377:dbl)  [unwired: 3 in, 1 out]
            n145 = Fract/Exp String To Number(string=w380) -> (number=w379:dbl)  [unwired: 3 in, 1 out]
          }
          frame #2 {
            n146 = case shown="False" "LI 3" {
              tunnel: [w393 w395] -> w390
              tunnel: [w393 w394] -> w391
              frame #0 {
                w393 = "0" ("Antwort1")
              }
              frame #1 {
                n147 = call "LI-Ansteuerung.vi"("Frage2"="OUTP? 4", "Frage1"="OUTP? 1", "address string"="GPIB L 3") -> ("Antwort2"=w395:string, "Antwort1"=w394:string)
              }
            }
            n148 = Fract/Exp String To Number(string=w391) -> (number=w389:dbl)  [unwired: 3 in, 1 out]
            n149 = Fract/Exp String To Number(string=w390) -> (number=w388:dbl)  [unwired: 3 in, 1 out]
          }
          frame #3 {
            n150 = case shown="True" "LI 4" {
              tunnel: [w404 w406] -> w401
              tunnel: [w404 w405] -> w402
              frame #0 {
                w404 = "0" ("Antwort1")
              }
              frame #1 {
                n151 = call "LI-Ansteuerung.vi"("Frage2"="OUTP? 4", "Frage1"="OUTP? 1", "address string"="GPIB L 4") -> ("Antwort2"=w406:string, "Antwort1"=w405:string)
              }
            }
            n152 = Fract/Exp String To Number(string=w401) -> (number=w399:dbl)  [unwired: 3 in, 1 out]
            n153 = Fract/Exp String To Number(string=w402) -> (number=w400:dbl)  [unwired: 3 in, 1 out]
          }
          frame #4 {
            n154 = case shown="True" "HP 1" {
              tunnel: [0.0 ("Voltage") w414] -> w410
              frame #0 {
              }
              frame #1 {
                n155 = call "HP-ReadVoltagev2.vi"("String"="meas:volt:dc? 200,0.001", "HP-Mulitmeter\nGPIB Address"="GPIB HP") -> ("Voltage"=w414:dbl)  [unwired: 9 in]
              }
            }
          }
          frame #5 {
            n156 = Get Date/Time In Seconds() -> (seconds since 1Jan1904=w417:timestamp)
            n157 = To Double Precision Float(number=w417) -> (double precision float=w416:dbl)
          }
        }
        n158 = Build Array(w356, w355, w354, w353, w350, w349, w347, w348, w346, w345, w344, w343) -> (w342:dbl[])
        n159 = Array To Spreadsheet String(array=w342, 3:"%f" ("format string")) -> (spreadsheet string=w352:string)  [unwired: 1 in]
        n160 = local read "Messfile Refnum"() -> (w358:refnum<file>)
        n161 = Set File Position(refnum=w358, from (0:start)=1, error in=w361) -> (refnum out=w360:refnum<file>, error out=w362:errorcluster)  [unwired: 1 in]
        n162 = Write to Text File(file (use dialog)=w360, text=w352, error in=w362) -> (refnum out=w364:refnum<file>, error out=w363:errorcluster)  [unwired: 1 in, 1 out]
        n163 = Flush File(refnum=w364, error in=w363) -> (error out=w357:errorcluster)  [unwired: 1 out]
      }
      frame #3 {
        n164 = local read "measured data"() -> (w423:dbl[][])
        n165 = Insert Into Array(array=w423, new element=w422) -> (w421:dbl[][])  [unwired: 2 in]
        n166 = case shown="0, Default" w420 {
          tunnel: w421 -> [w439 w453]
          tunnel: "Y Axis" -> [w441 w452]
          tunnel: "X Axis" -> [w427 w451]
          frame #0 {
            n167 = Index Array(array=w439, index (col)=1 ("disabled index (col)")) -> (element=w434:dbl[])  [unwired: 1 in]
            n168 = Index Array(array=w439, index (col)=0 ("disabled index (col)")) -> (element=w433:dbl[])  [unwired: 1 in]
            n169 = Square(x=w434) -> (x^2=w436:dbl[])
            n170 = Square(x=w433) -> (x^2=w437:dbl[])
            n171 = Index Array(array=w439, index (col)=w441) -> (element=w426:dbl[])  [unwired: 1 in]
            n172 = Divide(x=w434, y=w433) -> (x/y=w432:dbl[])
            n173 = Add(x=w437, y=w436) -> (x+y=w435:dbl[])
            n174 = Tangent(1:w432) -> (0:w431:dbl[])
            n175 = Square Root(x=w435) -> (sqrt(x)=w424:dbl[])
            n176 = Divide(x=w431, y=3.141592653589793) -> (x/y=w429:dbl[])
            n177 = Multiply(x=w429, y=180) -> (x*y=w425:dbl[])
            n178 = case shown="\"B\", Default" w427 {
              tunnel: w426 -> [w444 w447]
              tunnel: w425 -> [_ w446]
              tunnel: w424 -> [w443 _]
              frame #0 {
                n179 = Bundle(w443, "measured data"=w444) -> (w442:cluster{dbl[], "measured data":dbl[]})  [unwired: 1 in]
                n180 = local write "XY Graph"(w442) -> ()
              }
              frame #1 {
                n181 = Bundle(w446, "measured data"=w447) -> (w445:cluster{dbl[], "measured data":dbl[]})  [unwired: 1 in]
                n182 = local write "XY Graph"(w445) -> ()
              }
            }
          }
          frame #1 {
            n183 = Index Array(array=w453, index (col)=w451) -> (element=w450:dbl[])  [unwired: 1 in]
            n184 = Index Array(array=w453, index (col)=w452) -> (element=w449:dbl[])  [unwired: 1 in]
            n185 = Bundle("measured data"=w450, "measured data"=w449) -> (w448:T2)  [unwired: 1 in]
            n186 = local write "XY Graph"(w448) -> ()
          }
        }
        n187 = local write "measured data"(w421) -> ()
      }
    }
    n188 = local read "Ramping Control"() -> (w251:u16)
    n189 = case shown="1" w251 {
      selector: w251 -> [w455 w469 w487 w491 w506]
      tunnel: w250 -> [_ w472 _ w494 w511]
      tunnel: w249 -> [_ w471 _ w493 w510]
      tunnel: [w454 w470 w486 w492 w509] -> w248
      tunnel: [w455 w469 w487 w491 w506] -> w246
      tunnel: w245 -> [_ _ _ w490 w508]
      tunnel: w244 -> [_ _ _ _ w505]
      tunnel: w243 -> [_ _ _ _ w504]
      tunnel: w242 -> [_ w461 _ _ _]
      tunnel: w241 -> [w454 w457 w486 w488 w503]
      frame #0 {
      }
      frame #1 {
        w464 = T9."HOLDING" ("y")
        n190 = local read "Number of lines"() -> (w458:i32)
        n191 = local read "Starting index"() -> (w460:i32)
        n192 = call <userlib>:"Get Ramping Mode.vi"("Communications Config"=w472, "error in"=w457) -> ("Ramping Mode"=w467:T10, "error out"=w468:T5)  [unwired: 1 out]
        n193 = call <userlib>:"Get Ramping Mode.vi"("Communications Config"=w471, "error in"=w468) -> ("Ramping Mode"=w466:T10, "error out"=w470:T5)  [unwired: 1 out]
        n194 = Less?(x=w460, y=w458) -> (x < y?=w459:bool)
        n195 = Equal?(x=w467, y=w464) -> (x = y?=w463:bool)
        n196 = Equal?(x=w466, y=w464) -> (x = y?=w462:bool)
        n197 = Compound Arithmetic op=AND(w463, w462) -> (w465:bool)
        n198 = case shown="True" w465 {
          tunnel: w461 -> [_ w475]
          tunnel: w459 -> [_ w474]
          tunnel: "Wait between \nVectors (ms)" -> [_ w473]
          frame #0 {
          }
          frame #1 {
            n199 = case shown="1" w475 {
              tunnel: w474 -> [_ w479]
              tunnel: w473 -> [_ w478]
              frame #0 {
                w477 = u16 2 items=["NEXT VECTOR", "RAMPING", "HOLDING", "PAUSE", "ZERO"] ("Ramping Control")
                n200 = local write "STATUS"("Holding at current vector. Set Ramping Mode to NEXT VECTOR to continue." ("STATUS")) -> ()
                n201 = local write "Ramping Control"(w477) -> ()
              }
              frame #1 {
                # "Go to NEXT VECTOR automatically"
                n202 = case shown="True" w479 {
                  tunnel: w478 -> [_ w482]
                  frame #0 {
                    w481 = u16 2 items=["NEXT VECTOR", "RAMPING", "HOLDING", "PAUSE", "ZERO"] ("Ramping Control")
                    n203 = local write "STATUS"("Holding at current vector. Set Ramping Mode to NEXT VECTOR to continue." ("STATUS")) -> ()
                    n204 = local write "Ramping Control"(w481) -> ()
                  }
                  frame #1 {
                    n205 = stacked-sequence {
                      tunnel: w482 -> [w483 _]
                      frame #0 {
                        n206 = Wait (ms)(milliseconds to wait=w483) -> ()  [unwired: 1 out]
                      }
                      frame #1 {
                        w485 = u16 0 items=["NEXT VECTOR", "RAMPING", "HOLDING", "PAUSE", "ZERO"] ("Ramping Control")
                        n207 = local write "Ramping Control"(w485) -> ()
                        n208 = local write "STATUS"("Go to NEXT VECTOR" ("STATUS")) -> ()
                      }
                    }
                  }
                }
              }
            }
          }
        }
      }
      frame #2 {
      }
      frame #3 {
        n209 = Not Equal?(x=w491, y=w490) -> (x != y?=w489:bool)
        n210 = case shown="False" w489 {
          tunnel: w494 -> [_ w502]
          tunnel: w493 -> [_ w501]
          tunnel: [w495 w499] -> w492
          tunnel: w488 -> [w495 w496]
          frame #0 {
          }
          frame #1 {
            w497 = u16 1 items=["RAMP", "PAUSE", "MANUAL UP", "MANUAL DOWN", "ZERO"] ("Ramping Mode")
            n211 = call <userlib>:"Set Ramping Mode.vi"("error in"=w496, "Ramping Mode"=w497, "Communications Config"=w502) -> ("error out"=w500:T5)
            n212 = call <userlib>:"Set Ramping Mode.vi"("error in"=w500, "Ramping Mode"=w497, "Communications Config"=w501) -> ("error out"=w499:T5)
            n213 = local write "STATUS"("All Programmers are PAUSED. Set Ramping Mode to NEXT VECTOR to continue." ("STATUS")) -> ()
          }
        }
      }
      frame #4 {
        n214 = Not Equal?(x=w506, y=w508) -> (x != y?=w507:bool)
        n215 = case shown="False" w507 {
          tunnel: w511 -> [_ w520]
          tunnel: w510 -> [_ w519]
          tunnel: [w512 w515] -> w509
          tunnel: w505 -> [_ w518]
          tunnel: w504 -> [_ w517]
          tunnel: w503 -> [w512 w513]
          frame #0 {
          }
          frame #1 {
            w514 = u16 4 items=["RAMP", "PAUSE", "MANUAL UP", "MANUAL DOWN", "ZERO"] ("Ramping Mode")
            n216 = local write "STATUS"("Zeroing vector." ("STATUS")) -> ()
            n217 = call <userlib>:"Set Ramping Mode.vi"("error in"=w513, "Ramping Mode"=w514, "Communications Config"=w520) -> ("error out"=w523:T5)
            n218 = call <userlib>:"Set Ramping Mode.vi"("error in"=w523, "Ramping Mode"=w514, "Communications Config"=w519) -> ("error out"=w516:T5)
            n219 = call <userlib>:"Set Current Ramp Rate.vi"("Communications Config"=w520, "Ramp Rate (A/sec)"=w518, "error in"=w516) -> ("error out"=w521:T5)  [unwired: 2 in]
            n220 = call <userlib>:"Set Current Ramp Rate.vi"("Communications Config"=w519, "Ramp Rate (A/sec)"=w517, "error in"=w521) -> ("error out"=w515:T5)  [unwired: 2 in]
          }
        }
      }
    }
    n221 = local read "Continue Execution?"() -> (w247:bool)
    n222 = Wait Until Next ms Multiple(millisecond multiple=u32 100) -> ()  [unwired: 1 out]
  }
  n223 = case shown="0, Default" w29 {
    tunnel: w25 -> [w526 _ _]
    tunnel: w23 -> [w525 w529 w530]
    tunnel: [w524 w528 w530] -> w30
    tunnel: w24 -> [_ w527 _]
    frame #0 {
      n224 = call <userlib>:"430_TCP_Close.vi"("error in (no error)"=w525, "connection ID"=w526) -> ("error out"=w524:errorcluster)  [unwired: 1 out]
    }
    frame #1 {
      n225 = call <userlib>:"430_RS232_Close.vi"("error in (no error)"=w529, "VISA resource name"=w527) -> ("error out"=w528:errorcluster)  [unwired: 1 in]
    }
    frame #2 {
    }
  }
  n226 = case shown="0, Default" w28 {
    tunnel: w27 -> [w533 _ _]
    tunnel: w30 -> [w532 w536 w537]
    tunnel: [w531 w535 w537] -> w20
    tunnel: w26 -> [_ w534 _]
    frame #0 {
      n227 = call <userlib>:"430_TCP_Close.vi"("error in (no error)"=w532, "connection ID"=w533) -> ("error out"=w531:errorcluster)  [unwired: 1 out]
    }
    frame #1 {
      n228 = call <userlib>:"430_RS232_Close.vi"("error in (no error)"=w536, "VISA resource name"=w534) -> ("error out"=w535:errorcluster)  [unwired: 1 in]
    }
    frame #2 {
    }
  }
  "error out" <- w20
  n229 = local read "Magnetic Field Units"() -> (w47:u16)
  n230 = local read "Coordinate System"() -> (w48:u16)
  n231 = while {
    tunnel: "Starting index" -> [w545]
    tunnel: w22 -> [w551]
    tunnel: w21 -> [w552]
    tunnel: w47 -> [w553]
    tunnel: w48 -> [w554]
    tunnel: w45 -> [w557]
    tunnel: "Max Ramp Rate - Y Axis (A/s)" -> [w541]
    tunnel: "Max Ramp Rate - Z Axis (A/s)" -> [w540]
    tunnel: "Magnitude Limit (kG)" -> [w542]
    tunnel: "User defined Ramp Rate (T/min)" -> [w539]
    tunnel: "User defined Ramp Rate (T/min)" -> [w538]
    i -> [w544]
    stop <- w546 continue-if-true
    n232 = local read "Field Values"() -> (w548:string[][])
    n233 = Add(x=w545, y=w544) -> (x+y=w543:i32)
    n234 = while "Wait for NEXT VECTOR setting by operator." {
      tunnel: [w561] -> w556
      tunnel: w557 -> [w561]
      stop <- w562 continue-if-true
      w560 = u16 0 items=["NEXT VECTOR", "RAMPING", "HOLDING", "PAUSE", "ZERO"] ("Ramping Control")
      n235 = local read "Ramping Control"() -> (w563:u16)
      n236 = Not Equal?(x=w560, y=w563) -> (x != y?=w562:bool)
    }
    n237 = stacked-sequence {
      tunnel: w543 -> [w565 _ w571 _]
      frame #0 {
        (unwired) -2
        n238 = Subtract(x=w565, y=2) -> (x-y=w568:i32)
        n239 = Bundle(w568, -2) -> (w566:cluster{i32, i32})  [unwired: 1 in]
        n240 = property on="Field Values" class="Tbl (strict)"("Active Cell:Active Cell"=w566) -> ()  [unwired: 2 in, 2 out]
      }
      frame #1 {
        n241 = local read "Normal color"() -> (w569:u32)
        n242 = property on="Field Values" class="Tbl (strict)"("Active Cell:Cell Background Color"=w569) -> ()  [unwired: 2 in, 2 out]
      }
      frame #2 {
        n243 = Decrement(x=w571) -> (x-1=w570:i32)
        n244 = Bundle(w570, -2) -> (w573:cluster{i32, i32})  [unwired: 1 in]
        n245 = property on="Field Values" class="Tbl (strict)"("Active Cell:Active Cell"=w573) -> ()  [unwired: 2 in, 2 out]
      }
      frame #3 {
        n246 = property on="Field Values" class="Tbl (strict)"("Active Cell:Cell Background Color"="Highlight color") -> ()  [unwired: 2 in, 2 out]
      }
    }
    n247 = Index Array(array=w548, index (row)=w543) -> (element=w555:string[])  [unwired: 1 in]
    n248 = local write "Starting index"(w543) -> ()
    n249 = Add(x=1, y=w543) -> (x+y=w558:i32)
    n250 = Number To Decimal String(number=w558) -> (decimal integer string=w547:string)  [unwired: 1 in]
    n251 = stacked-sequence {
      tunnel: [_ w599] -> w549
      tunnel: [_ w598] -> w550
      tunnel: w556 -> [_ w594]
      tunnel: w555 -> [_ w593]
      tunnel: w554 -> [_ w592]
      tunnel: w553 -> [_ w591]
      tunnel: w552 -> [_ w590]
      tunnel: w551 -> [_ w589]
      tunnel: w547 -> [_ w588]
      tunnel: w542 -> [_ w586]
      tunnel: w541 -> [_ w585]
      tunnel: w540 -> [_ w580]
      tunnel: w539 -> [_ w584]
      tunnel: w538 -> [_ w583]
      frame #0 {
        w578 = u16 1 items=["NEXT VECTOR", "RAMPING", "HOLDING", "PAUSE", "ZERO"] ("Ramping Control")
        n252 = local write "Ramping Control"(w578) -> ()
      }
      frame #1 {
        n253 = call <userlib>:"Set 2D Next Vector_entwurf.vi"("Coordinate System"=w592, "Magnetic Field Units"=w591, 3:"User defined Ramp Rate (T/min)"=w583, "Magnitude Limit (kG)"=w586, "Y-Axis Communications Config"=w590, "Input Vector"=w593, "Z-Axis Communications Config"=w589, 10:"User defined Ramp Rate (T/min)"=w584, "Max Ramp Rate - Y Axis (A/s)"=w585, "error in"=w594, "Max Ramp Rate - Z Axis (A/s)"=w580) -> ("Y-Axis Ramp Rate (T/min)"=→"Current Ramp Rate Y (T/min)":dbl, "Within Limits?"=w599:bool, "Ramp Rate along Vector (T/min)"=→"Ramp Rate along Vector (T/min)":dbl, "Z-Axis Ramp Rate (T/min)"=→"Current Ramp Rate Z (T/min)":dbl, "All Instruments Responded?"=w598:bool, "error out"=w587:T5)  [unwired: 3 in]
        n254 = Concatenate Strings("Ramping to field vector " ("STATUS"), w588, "..." ("STATUS")) -> (w595:string)
        n255 = local write "error in"(w587) -> ()
        n256 = local write "STATUS"(w595) -> ()
      }
    }
    n257 = case shown="True" w549 {
      tunnel: w550 -> [_ w576]
      frame #0 {
        n258 = local write "STATUS"("Vector magnitude limt or maximum coil current exceeded. Vector ignored. VI halted." ("STATUS")) -> ()
      }
      frame #1 {
        n259 = case shown="True" w576 {
          frame #0 {
            n260 = local write "STATUS"("Not all programmers responded. VI halted." ("STATUS")) -> ()
          }
          frame #1 {
          }
        }
      }
    }
    n261 = Compound Arithmetic op=AND(w550, w549) -> (w546:bool)
    n262 = local write "Continue Execution?"(w546) -> ()
  }
